vi "Write Data.vi"(6 "Data":T1(array[cluster]), 11 "Handle Drag Starting Msg in":refnum<class "Handle Drag Starting Msg.lvclass">) -> (3 "Handle Drag Starting Msg out":refnum<class "Handle Drag Starting Msg.lvclass">)   [LabVIEW 2019, in "File Explorer.lvlib" / "Handle Drag Starting Msg.lvclass"]
uses:
  <vilib>/gpm_packages/@cs/file-explorer-extension/Source/File Explorer/File Explorer Messages/Handle Drag Starting Msg/Handle Drag Starting Msg.lvclass
  <vilib>/gpm_packages/@cs/file-explorer-extension/Source/File Explorer/File Explorer Messages/Handle Drag Starting Msg/Handle Drag Starting Msg.lvclass/Handle Drag Starting Msg.ctl
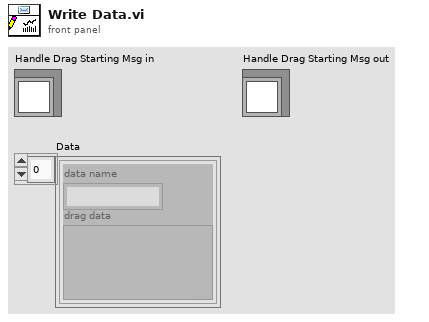
[diagram p1: front panel]
types:
  T1 = cluster{"data name":string, "drag data":variant}[]
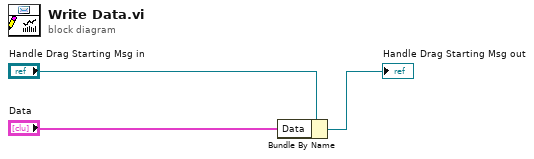
[diagram p0: block diagram]
diagram:
  n1 = Bundle By Name(cluster="Handle Drag Starting Msg in", "Data"="Data") -> (→"Handle Drag Starting Msg out":refnum<class "Handle Drag Starting Msg.lvclass">)
